vi "FIRE_MULTIPLE.vi"(10 "argv":string[](array[string]), 11 "args":u8) -> ()   [LabVIEW 2011]
uses:
  <vilib>/Rock Robotics/WPI/DriverStation/WPI_DriverStationStatusErrorCache.ctl
  signals/Signal.ctl
  Auto_Conf.vi
panel:
  in  "shot_interval":u32=1200
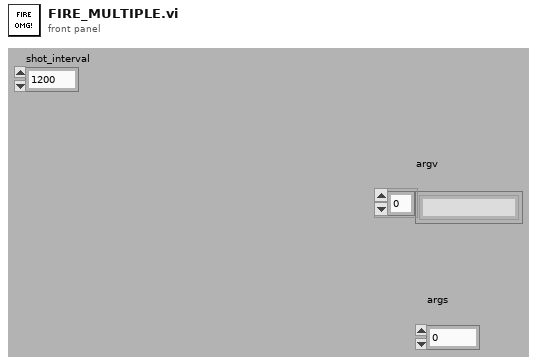
[diagram p1: front panel]
types:
  T1 = typedef "WPI_DriverStationStatusErrorCache.ctl" = enum16{"Get", "Set"}
  T2 = typedef "Signal.ctl" = enum16{"SIGFIRE", "SIGSTOPSCRIPT", "SIGSTARTGUN", "SIGSTOPGUN", "SIGDISABLED", "SIGENABLED", "SIGUDPTIMEOUT", "SIGNEWVISION_REMOTE", "SIGNEWVISION_LOCAL", "SIGSHOTFIRED", "SIGDOTRACK", "SIGDONTTRACK"}
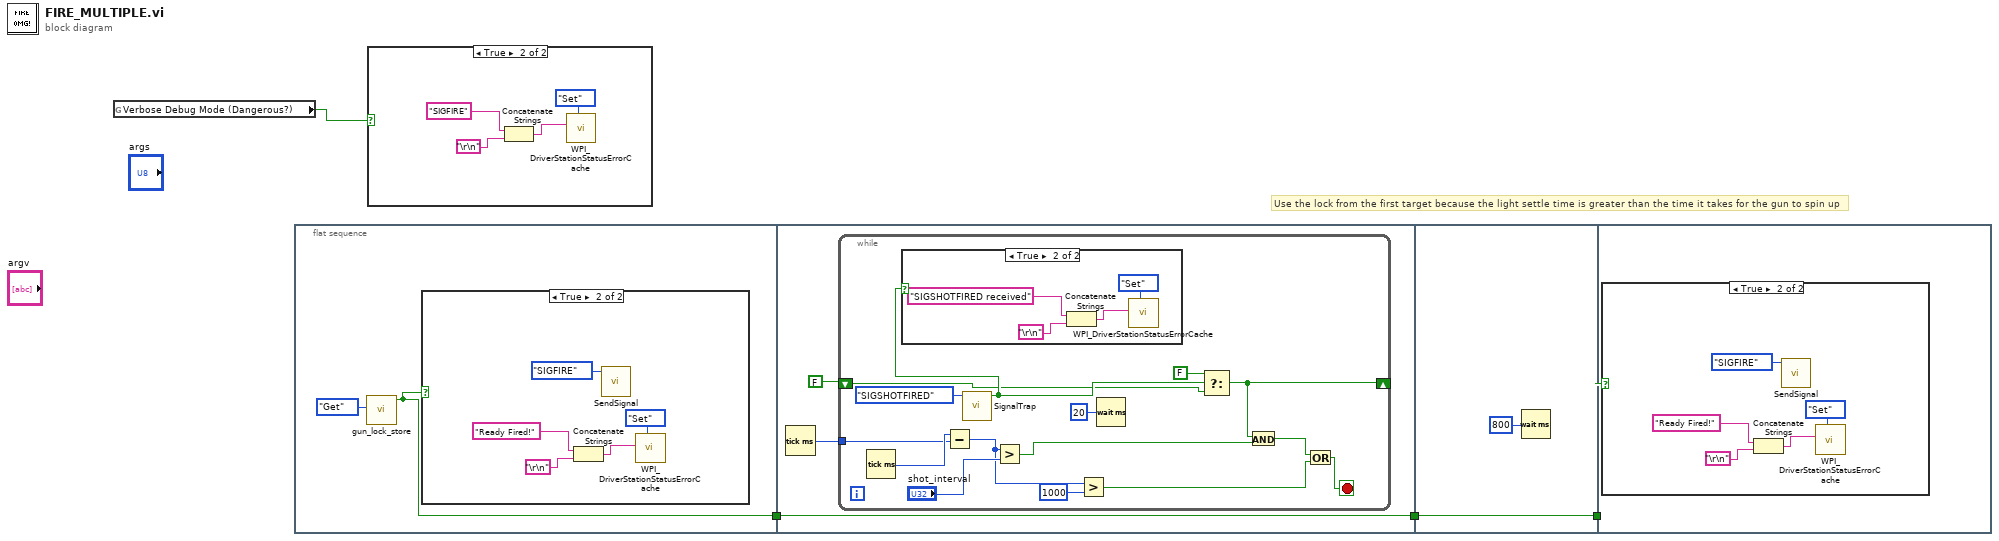
[diagram p0: block diagram]
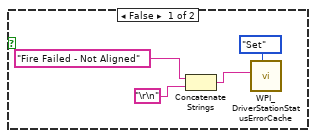
[diagram p2: hidden frame]
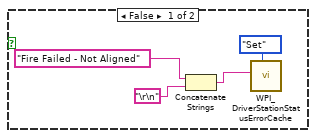
[diagram p4: hidden frame]
diagram:
  # "Use the lock from the first target because the light settle time is greater than the time it takes for the gun to spin up"
  n1 = global read "Auto_Conf.vi" "Verbose Debug Mode (Dangerous?)"() -> (w4:bool)
  n2 = flat-sequence {
    tunnel: [w5] -> w3
    tunnel: w3 -> [w16]
    tunnel: [w16] -> w2
    tunnel: w2 -> [w39]
    tunnel: [w39] -> w1
    tunnel: w1 -> [w40]
    frame #0 {
      n3 = call "gun_lock_store.vi"("data_store_mode"=enum16{"Set", "Get"}."Get") -> ("Lock"=w5:bool)  [unwired: 10 in]
      n4 = case shown="True" w5 {
        frame False {
          n5 = Concatenate Strings("Fire Failed - Not Aligned" ("string"), "\r\n") -> (w8:string)
          n6 = call <vilib>:"WPI_DriverStationStatusErrorCache.vi"("StatusErrorCacheOp"=WPI_DriverStationStatusErrorCache."Set", "Error String"=w8) -> ()  [unwired: 10 out]
        }
        frame True {
          n7 = Concatenate Strings("Ready Fired!" ("string"), "\r\n") -> (w13:string)
          n8 = call "SendSignal.vi"("Signal"=Signal."SIGFIRE") -> ()  [unwired: 11 in]
          n9 = call <vilib>:"WPI_DriverStationStatusErrorCache.vi"("StatusErrorCacheOp"=WPI_DriverStationStatusErrorCache."Set", "Error String"=w13) -> ()  [unwired: 10 out]
        }
      }
    }
    frame #1 {
      n10 = Tick Count (ms)() -> (millisecond timer value=w18:u32)
      n11 = while {
        tunnel: w18 -> [w31]
        shift-right: [w22] -> _
        shift-left: FALSE -> [w26]
        stop <- w29 stop-if-true
        n12 = Tick Count (ms)() -> (millisecond timer value=w32:u32)
        n13 = Subtract(x=w32, y=w31) -> (x-y=w24:u32)
        n14 = call "SignalTrap.vi"("Signal"=Signal."SIGSHOTFIRED") -> ("Trapped Signal"=w27:bool)  [unwired: 10 in]
        n15 = case shown="True" w27 {
          frame False {
          }
          frame True {
            n16 = Concatenate Strings("SIGSHOTFIRED received" ("string"), "\r\n") -> (w36:string)
            n17 = call <vilib>:"WPI_DriverStationStatusErrorCache.vi"("StatusErrorCacheOp"=WPI_DriverStationStatusErrorCache."Set", "Error String"=w36) -> ()  [unwired: 10 out]
          }
        }
        n18 = Greater?(x=w24, y="shot_interval") -> (0:w21:bool)
        n19 = Greater?(x=w24, y=u32 1000) -> (0:w19:bool)
        n20 = Wait (ms)(milliseconds to wait=u32 20) -> ()  [unwired: 1 out]
        n21 = Select(t=FALSE, s=w27, f=w26) -> (s? t:f=w22:bool)
        n22 = And(x=w22, y=w21) -> (x .and. y?=w20:bool)
        n23 = Or(x=w20, y=w19) -> (x .or. y?=w29:bool)
      }
    }
    frame #2 {
      n24 = Wait (ms)(milliseconds to wait=u32 800) -> ()  [unwired: 1 out]
    }
    frame #3 {
      n25 = case shown="True" w40 {
        frame False {
          n26 = Concatenate Strings("Fire Failed - Not Aligned" ("string"), "\r\n") -> (w42:string)
          n27 = call <vilib>:"WPI_DriverStationStatusErrorCache.vi"("StatusErrorCacheOp"=WPI_DriverStationStatusErrorCache."Set", "Error String"=w42) -> ()  [unwired: 10 out]
        }
        frame True {
          n28 = Concatenate Strings("Ready Fired!" ("string"), "\r\n") -> (w47:string)
          n29 = call "SendSignal.vi"("Signal"=Signal."SIGFIRE") -> ()  [unwired: 11 in]
          n30 = call <vilib>:"WPI_DriverStationStatusErrorCache.vi"("StatusErrorCacheOp"=WPI_DriverStationStatusErrorCache."Set", "Error String"=w47) -> ()  [unwired: 10 out]
        }
      }
    }
  }
  n31 = case shown="True" w4 {
    frame False {
    }
    frame True {
      n32 = Concatenate Strings("SIGFIRE" ("string"), "\r\n") -> (w51:string)
      n33 = call <vilib>:"WPI_DriverStationStatusErrorCache.vi"("StatusErrorCacheOp"=WPI_DriverStationStatusErrorCache."Set", "Error String"=w51) -> ()  [unwired: 10 out]
    }
  }
